vi "Query Trace Data.vi"(8 "error in (no error)":errorcluster, 11 "MXA in":refnum<class "MXA.lvclass">) -> (0 "error out":errorcluster, 1 "Level":dbl[](array[numeric]), 2 "Frequency/Time":dbl[](array[numeric]), 3 "MXA out":refnum<class "MXA.lvclass">)   [LabVIEW 2020, in "MXA.lvclass"]
uses:
  MXA.lvclass
  C:/Sandbox/Git_Sandbox/WiSpry Test Framework source code (LV20)/WiSpry Test Framework/Instruments/Spectrum Analyzer/Spectrum Analyzer.lvclass
  C:/Sandbox/Git_Sandbox/WiSpry Test Framework source code (LV20)/WiSpry Test Framework/Instruments/Instrument.lvclass
  Instrument.lvclass/Instrument.ctl
  Spectrum Analyzer.lvclass/Spectrum Analyzer.ctl
  <instrlib>/Agilent MXA Series/Public/Data/Low Level/Fetch Trace (Swept SA).vi
  Instrument.lvclass
  <instrlib>/Agilent MXA Series/Agilent MXA Series.lvlib
  Spectrum Analyzer.lvclass
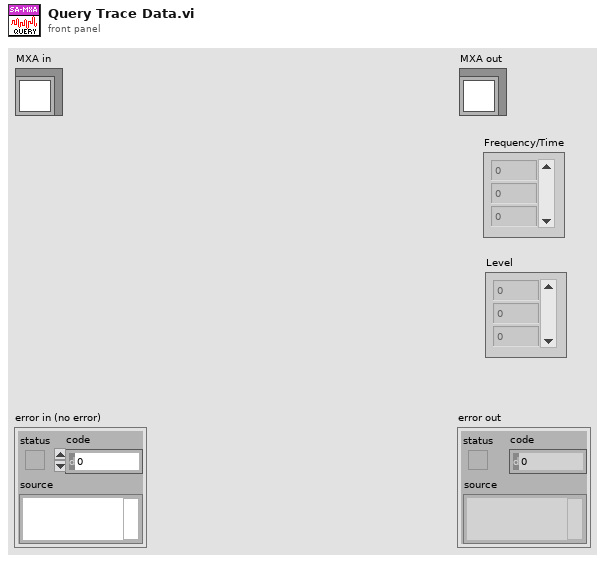
[diagram p1: front panel]
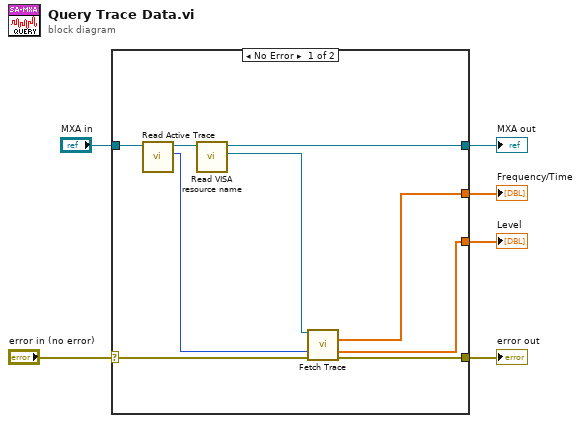
[diagram p0: block diagram]
diagram:
  n1 = case shown="No Error" "error in (no error)" {
    selector: "error in (no error)" -> [w14 w17]
    tunnel: "MXA in" -> [w7 w16]
    tunnel: [w12 w17] -> w5
    tunnel: [w15 w16] -> w3
    tunnel: [w11 _] -> w2
    tunnel: [w10 _] -> w1
    frame No Error {
      n2 = call "Read Active Trace.vi"("Spectrum Analyzer in"=w7) -> ("Active Trace"=w9:u16, "Spectrum Analyzer out"=w8:refnum<class "MXA.lvclass">)  [unwired: 9 in]
      n3 = call "Read VISA resource name.vi"("Instrument in"=w8) -> ("VISA resource name"=w13:refnum<visa-resource-name>, "Instrument out"=w15:refnum<class "MXA.lvclass">)  [unwired: 9 in]
      n4 = call-poly <instrlib>:"Fetch Trace.vi"("VISA resource name"=w13, "Trace Name (1: Trace 1)"=w9, "error in (no error)"=w14) -> ("X Array"=w10:dbl[], "Y Array"=w11:dbl[], "error out"=w12:errorcluster)  [unwired: 9 in, 1 out]
    }
    frame Error {
    }
  }
  "error out" <- w5
  "MXA out" <- w3
  "Level" <- w2
  "Frequency/Time" <- w1
